vi "Get Path Regex.vi"(8 "error in (no error)":errorcluster, 11 "Test HTTPS Controller in":refnum<class "Test HTTPS Controller.lvclass">) -> (0 "error out":errorcluster, 2 "Path Regex":string, 3 "Test HTTPS Controller out":refnum<class "Test HTTPS Controller.lvclass">)   [LabVIEW 2020, in "Test HTTPS Controller.lvclass"]
uses:
  Test HTTPS Controller.lvclass
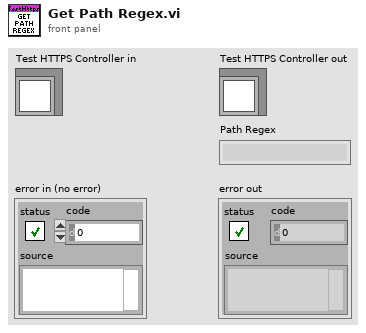
[diagram p1: front panel]
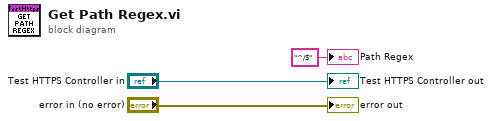
[diagram p0: block diagram]
diagram:
  "error out" <- "error in (no error)"
  "Test HTTPS Controller out" <- "Test HTTPS Controller in"
  "Path Regex" <- "^/$" ("Path Regex")
